vi "DOA (SubVI).vi"(8 "fix delay":dbl, 9 "sampling freq":dbl, 11 "delay array":dbl[](array[numeric])) -> (0 "fatal angle error?":bool, 1 "NaN?":bool, 2 "average angle":dbl, 3 "angles":dbl[](array[numeric]), 4 "angle error?":bool, 5 "sample delay":dbl[](array[numeric]))   [LabVIEW 2017]
doc: "Vi przekształca informację o opóźnieniu pomiędzy \"maksimami\" sygnałów na kąt padania dźwięku."
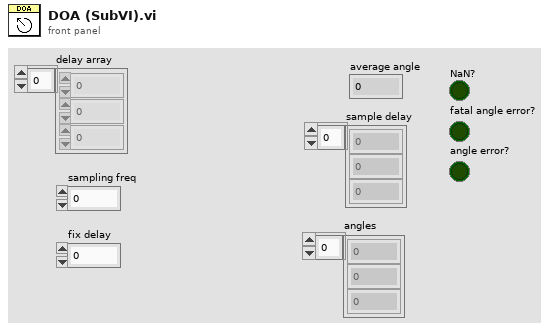
[diagram p1: front panel]
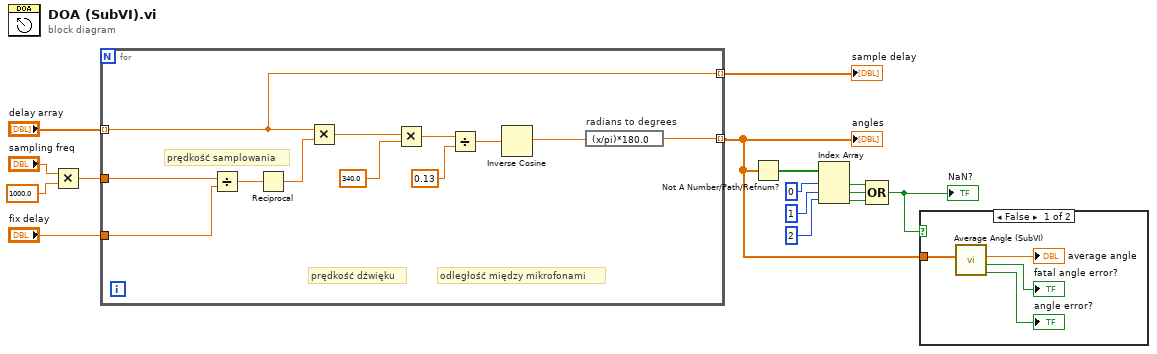
[diagram p0: block diagram]
diagram:
  n1 = Multiply(x="sampling freq", y=1000.0) -> (x*y=w12:dbl)
  n2 = for {
    tunnel: "delay array" -> [w21] mode=indexing
    tunnel: [w22] -> w1 mode=indexing
    tunnel: [w21] -> w15 mode=indexing
    tunnel: "fix delay" -> [w18]
    tunnel: w12 -> [w16]
    # "prędkość samplowania"
    # "odległość między mikrofonami"
    # "prędkość dźwięku"
    n3 = Divide(x=w16, y=w18) -> (x/y=w19:dbl)
    n4 = Reciprocal(x=w19) -> (1/x=w27:dbl)
    n5 = Multiply(x=w21, y=w27) -> (x*y=w23:dbl)
    n6 = Multiply(x=w23, y=340.0) -> (x*y=w25:dbl)
    n7 = Divide(x=w25, y=0.13) -> (x/y=w26:dbl)
    n8 = Inverse Cosine(1:w26) -> (0:w17:dbl)
    n9 = expression code="(x/pi)*180.0" "radians to degrees"(w17) -> (w22:dbl)
  }
  "angles" <- w1
  "sample delay" <- w15
  n10 = Not A Number/Path/Refnum?(number/path/refnum=w1) -> (NaN/Path/Refnum?=w9:bool[])
  n11 = Index Array(array=w9, index #1=0 ("index"), index #2=1 ("index"), index #3=2 ("index")) -> (element #1=w3:bool, element #2=w4:bool, element #3=w5:bool)
  n12 = Compound Arithmetic op=OR(w3, w4, w5) -> (w2:bool)
  "NaN?" <- w2
  n13 = case shown="False" w2 {
    tunnel: w1 -> [w30 _]
    frame False {
      n14 = call "Average Angle (SubVI).vi"("angles"=w30) -> ("average angle"=→"average angle":dbl, "fatal angle error?"=→"fatal angle error?":bool, "angle error?"=→"angle error?":bool)  [unwired: 7 in]
    }
    frame True {
    }
  }
